vi "ROI group-Rename ROI Group.vi"(7 "Save? (T)":bool=TRUE, 8 "error in (no error)":errorcluster, 9 "From clicked array element":bool, 10 "Index of renamed group":i32, 11 "Old group name":string) -> (0 "error out":errorcluster)   [LabVIEW 2020]
uses:
  Experiment header interface/Typedefs/Save-Load-Save as-Load last enum.ctl
  Global variables/gl_Functional Imaging-Global variables.vi
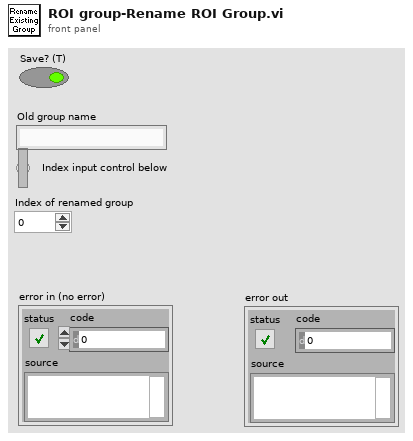
[diagram p1: front panel]
types:
  T1 = typedef "Functional Imging UI Refs.ctl" = cluster{"Menu ref":refnum<k9>, "Image control":refnum<vi>, "VI ref":refnum<vi>, "XGrapher":refnum<vi>, "Smoothing":refnum<vi>, "POI Averaging":refnum<vi>, "Normalize":refnum<vi>, "POI data points in each trial":refnum<vi>, "Channel":refnum<vi>, "Experiment data folder path":refnum<vi>, "[ROI vis]":refnum<vi>, "[Groups] visbl":T2, "Group Name":refnum<vi>, "POI index":refnum<vi>, "Trial No.":refnum<vi>, "Intensity Zoom":refnum<vi>, "Trial Cursor Enabled":refnum<vi>, "Number of Trials (ind 1)":refnum<vi>, "Number of Trials (ind 2)":refnum<vi>, "MiniScans Available":refnum<vi>, "POI Available":refnum<vi>, "Defer graph updates":refnum<vi>, "Waveform selector":refnum<vi>, "#of selected POI":refnum<vi>, "#of selected MiniScans":refnum<vi>, "#of selected groups":refnum<vi>, "Max Z-Projection":refnum<vi>, "Z-Plane Selector":refnum<vi>, "Index of miniscan point to visualise":refnum<vi>, "ROI vis. mode":refnum<vi>, "Total # of points":refnum<vi>, "Index of group clicked on":refnum<vi>, "Pane 1":refnum<vi>, "Pane 2":refnum<vi>, "Pane 3":refnum<vi>, "Pane 4":refnum<vi>, "Pane 5":refnum<vi>, "Pane 6":refnum<vi>, "Deselect all ROI":refnum<vi>, "Deselect all groups":refnum<vi>}
  T2 = typedef "Groups array referecne.ctl" = refnum<vi>
  T3 = typedef "Group sel cluster.ctl" = cluster{"Group number":string, "Group Name":string, "Visibility":bool, "Highlight":bool}
  T4 = typedef "Save-Load-Save as-Load last enum.ctl" = enum16{"Save file", "Save file as", "Load file", "Load last file"}
  T5 = typedef "ROI group info cluster.ctl" = cluster{"Group name":string, "# ROI in group":i32, "ROI numbers in group":i32[], "Group region specifier cluster":T6}
  T6 = typedef "ROI Descriptor" = cluster{"Global Rectangle":i32[], "Contours":cluster{"ID":enum32{"External", "Internal"}, "Type":u32, "Coordinates":i32[]}[]}
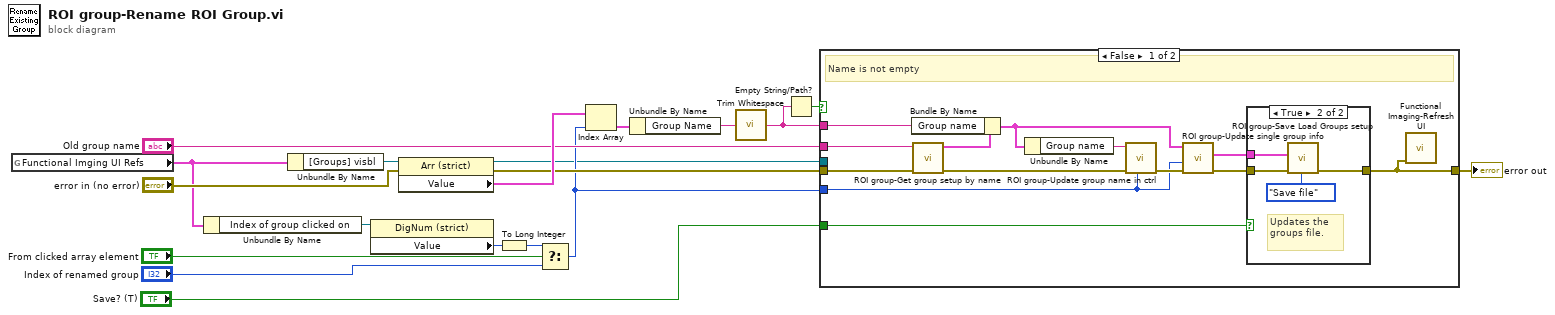
[diagram p0: block diagram]
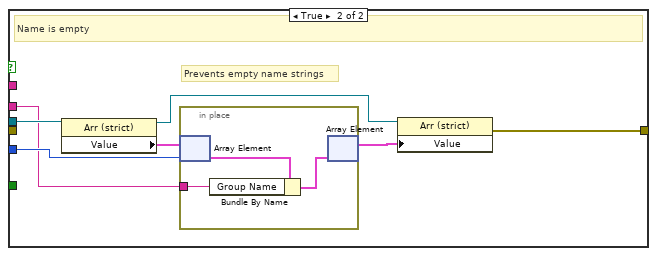
[diagram p3: hidden frame]
diagram:
  n1 = global read "gl_Functional Imaging-Global variables.vi" "Functional Imging UI Refs"() -> (w12:T1)
  n2 = Unbundle By Name(w12) -> ("Index of group clicked on"=w14:refnum<vi>)
  n3 = Unbundle By Name(w12) -> ("[Groups] visbl"=w19:T2)
  n4 = property on="Property Node" class="DigNum (strict)"(reference=w14) -> ("Value"=w13:i16)  [unwired: 1 in, 2 out]
  n5 = property on="Property Node" class="Arr (strict)"(reference=w19, error in="error in (no error)") -> (reference out=w2:T2, error out=w15:errorcluster, "Value"=w17:T3[])
  n6 = To Long Integer(number=w13) -> (32bit integer=w10:i32)
  n7 = Select(t=w10, s="From clicked array element", f="Index of renamed group") -> (s? t:f=w6:i32)
  n8 = Index Array(array=w17, index=w6) -> (element=w16:T3)
  n9 = Unbundle By Name(w16) -> ("Group Name"=w5:string)
  n10 = call <vilib>:"Trim Whitespace.vi"("string"=w5) -> ("trimmed string"=w3:string)  [unwired: 1 in]
  n11 = Empty String/Path?(string/path=w3) -> (empty?=w4:bool)
  n12 = case shown="False" w4 {
    tunnel: w15 -> [w32 _]
    tunnel: [w22 w38] -> w11
    tunnel: "Old group name" -> [w30 w41]
    tunnel: w3 -> [w26 _]
    tunnel: w6 -> [w24 w42]
    tunnel: w2 -> [_ w44]
    tunnel: "Save? (T)" -> [w20 _]
    frame False {
      # "Name is not empty"
      n13 = call "ROI group-Get group setup by name.vi"("error in"=w32, "Name of ROI group to search for"=w30) -> ("error out (no error)"=w31:errorcluster, "POI group info cluster"=w27:T5)  [unwired: 7 in, 1 out]
      n14 = Bundle By Name(cluster=w27, "Group name"=w26) -> (w25:T5)
      n15 = Unbundle By Name(w25) -> ("Group name"=w29:string)
      n16 = call "ROI group-Update group name in ctrl.vi"("Index of group to update"=w24, "error in (no error)"=w31, "Group Name"=w29) -> ("error out"=w28:errorcluster)  [unwired: 8 in]
      n17 = call "ROI group-Update single group info.vi"("error in (no error)"=w28, "Index of renamed group"=w24, "POI group info cluster"=w25) -> ("error out"=w21:errorcluster, "Updated \"All groups\" setup"=w23:T5[])  [unwired: 7 in]
      n18 = case shown="True" w20 {
        tunnel: w21 -> [w33 w36]
        tunnel: w23 -> [_ w35]
        tunnel: [w33 w34] -> w22
        frame False {
        }
        frame True {
          # "Updates the groups file."
          n19 = call "ROI group-Save Load Groups setup.vi"("error in (no error)"=w36, "Function"=Save-Load-Save_as-Load_last_enum."Save file", "Groups setup to save"=w35) -> ("error out"=w34:errorcluster)  [unwired: 7 in, 1 out]
        }
      }
      n20 = call "Functional Imaging-Refresh UI.vi"("error in (no error)"=w22) -> ()  [unwired: 11 in]
    }
    frame True {
      # "Prevents empty name strings"
      # "Name is empty"
      n21 = property on="Property Node" class="Arr (strict)"(reference=w44) -> (reference out=w40:T2, "Value"=w43:T3[])  [unwired: 1 in, 1 out]
      n22 = in-place {
        in-place-border: w41 -> [w45]
        n23 = in-place-array #1(w43, w42) -> (w47:T3)
        n24 = Bundle By Name(cluster=w47, "Group Name"=w45) -> (w46:T3)
        n25 = in-place-array #1(w46) -> (w39:T3[])  [unwired: 1 out]
      }
      n26 = property on="Property Node" class="Arr (strict)"(reference=w40, "Value"=w39) -> (error out=w38:errorcluster)  [unwired: 1 in, 1 out]
    }
  }
  "error out" <- w11
